vi "Sub_client_v1.vi"() -> ()   [LabVIEW 2019]
uses:
  <vilib>/LabVIEW Open Source Project/MQTT Client/Client class/Client.lvclass/Client.ctl
  <vilib>/LabVIEW Open Source Project/MQTT Connection/MQTT_Base/Base Class/MQTT_Base.lvclass/MQTT_Base.ctl
  <vilib>/LabVIEW Open Source Project/MQTT TCP Connection/MQTT_TCP/Connection/TCPConnection.lvclass
  C:/Program Files (x86)/National Instruments/LabVIEW 2019/vi.lib/LabVIEW Open Source Project/MQTT Connection/MQTT_Connection/Connection/Connection.lvclass
  <vilib>/LabVIEW Open Source Project/MQTT Client/Client class/Client.lvclass
  C:/Program Files (x86)/National Instruments/LabVIEW 2019/vi.lib/LabVIEW Open Source Project/MQTT Connection/MQTT_Base/Base Class/MQTT_Base.lvclass
  <vilib>/LabVIEW Open Source Project/MQTT Control Packets/Control Packets/PUBLISH/PUBLISH.lvclass
  <vilib>/LabVIEW Open Source Project/MQTT Connection/MQTT_Base/Base Class/MQTT_Base.lvclass
panel:
  out "Unsuback":bool
  out "Suback":bool
  in  "Subscribe":bool
  in  "Connection":bool
  in  "Stop Client":bool
  out "Waveform Chart":dbl(graph)
  out "last error":errorcluster
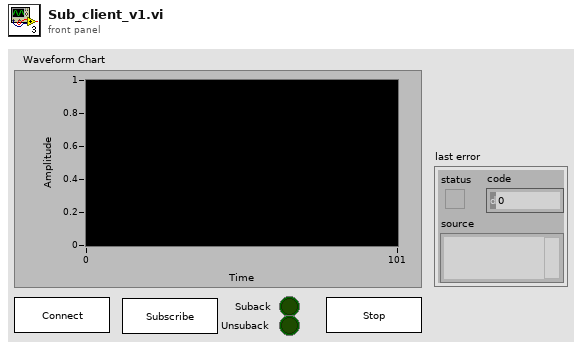
[diagram p1: front panel]
types:
  T1 = typedef "MQTT Client.lvlib/Client.lvclass/Public Events -- cluster.ctl" = cluster{"Connection Status":refnum<user-event>, "Connected":refnum<user-event>, "Application Message":refnum<user-event>}
  T2 = typedef "MQTT Base.lvlib/MQTT_Base.lvclass/Public Events -- cluster.ctl" = cluster{"Stop Event":refnum<user-event>, "Error Event":refnum<user-event>, "Inbound Message":refnum<user-event>}
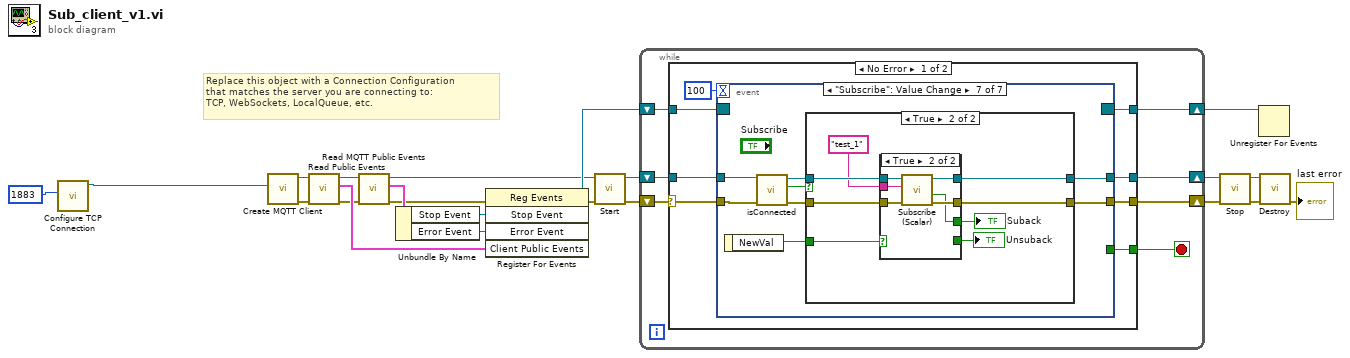
[diagram p0: block diagram]
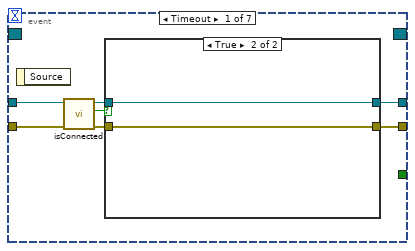
[diagram p2: hidden frame]
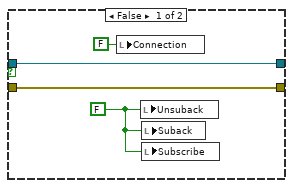
[diagram p3: hidden frame]
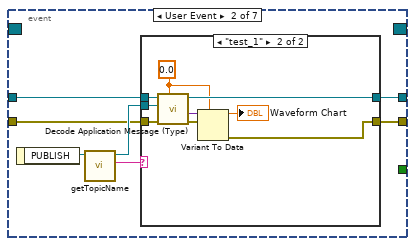
[diagram p4: hidden frame]
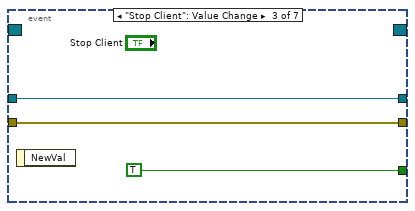
[diagram p6: hidden frame]
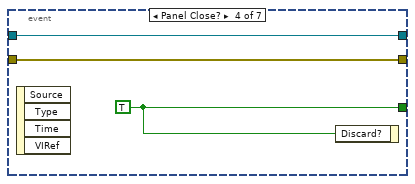
[diagram p7: hidden frame]
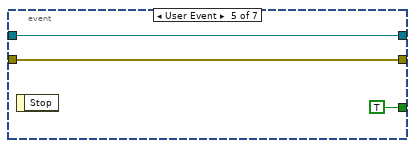
[diagram p8: hidden frame]
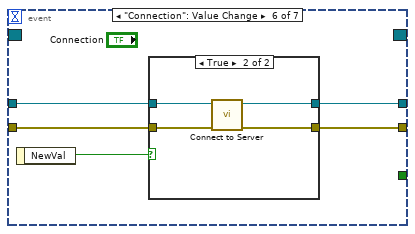
[diagram p9: hidden frame]
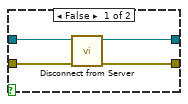
[diagram p10: hidden frame]
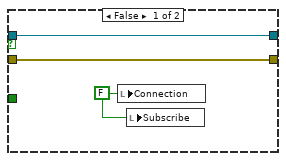
[diagram p11: hidden frame]
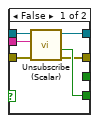
[diagram p12: hidden frame]
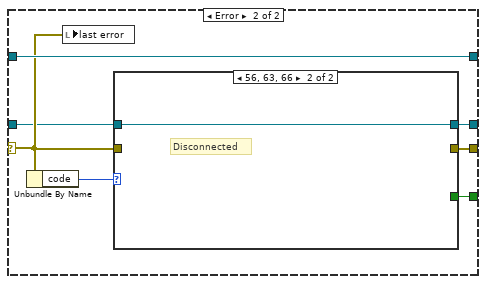
[diagram p13: hidden frame]
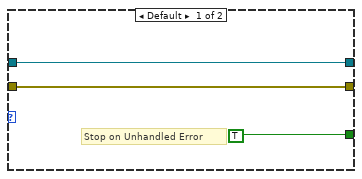
[diagram p14: hidden frame]
diagram:
  # "Replace this object with a Connection Configuration\nthat matches the server you are connecting to:\nTCP, WebSockets, LocalQueue, etc."
  n1 = call <vilib>:"Configure TCP Connection.vi"("remote port (80)"=u16 1883) -> ("TCPConnection"=w1:refnum<class "TCPConnection.lvclass">)  [unwired: 9 in, 1 out]
  n2 = call <vilib>:"Create MQTT Client.vi"("Connection Configuration"=w1) -> ("error out"=w5:errorcluster, "Client out"=w3:refnum<class "Client.lvclass">)  [unwired: 9 in]
  n3 = call <vilib>:"Read Public Events.vi"("error in (no error)"=w5, "Client in"=w3) -> ("error out"=w6:errorcluster, "Client Public Events"=w8:T1, "Client out"=w4:refnum<class "Client.lvclass">)  [unwired: 7 in]
  n4 = call <vilib>:"Read MQTT Public Events.vi"("error in (no error)"=w6, "MQTT_Base in"=w4) -> ("error out"=w7:errorcluster, "MQTT Public Events"=w15:T2, "MQTT_Base out"=w10:refnum<class "Client.lvclass">)  [unwired: 7 in]
  n5 = Unbundle By Name(w15) -> ("Stop Event"=w13:refnum<user-event>, "Error Event"=w14:refnum<user-event>)
  n6 = register-events(error in=w7, w13, w14, w8) -> (reference out=w11:refnum<event-registration>, error out=w9:errorcluster)  [unwired: 1 in]
  n7 = call <vilib>:"Start.vi"("error in (no error)"=w9, "MQTT_Base in"=w10) -> ("error out"=w21:errorcluster, "MQTT_Base out"=w20:refnum<class "Client.lvclass">)  [unwired: 7 in, 1 out]
  n8 = while {
    shift-right: [w28] -> w12
    shift-left: w11 -> [w29]
    shift-right: [w25] -> w17
    shift-left: w20 -> [w26]
    shift-right: [w27] -> w19
    shift-left: w21 -> [w23]
    stop <- w24 stop-if-true
    n9 = case shown="No Error" w23 {
      selector: w23 -> [w30 w125]
      tunnel: w29 -> [w37 w128]
      tunnel: [w36 w128] -> w28
      tunnel: [w35 w123] -> w27
      tunnel: w26 -> [w33 w124]
      tunnel: [w32 w127] -> w25
      tunnel: [w31 w122] -> w24
      frame No Error {
        n10 = event shown="[6] \"Subscribe\": Value Change" {
          selector: w37 -> [_ _ _ _ _ _ _]
          dyn-events: [_ _ _ _ _ _ _] -> w36
          timeout: 100 -> [_ _ _ _ _ _ _]
          tunnel: w30 -> [w40 w54 w70 w72 w77 w78 w96]
          tunnel: [w43 w51 w70 w72 w77 w79 w97] -> w35
          tunnel: [_ _ TRUE w74 TRUE _ _] -> w31
          tunnel: w33 -> [w42 w55 w71 w73 w75 w82 w95]
          tunnel: [w44 w53 w71 w73 w75 w80 w98] -> w32
          event Timeout {
            n11 = event-data() -> ()  [unwired: 1 in, 1 out]
            n12 = call <vilib>:"isConnected.vi"("error in (no error)"=w40, "Client in"=w42) -> ("error out"=w39:errorcluster, "connected"=w38:bool, "Client out"=w41:refnum<class "Client.lvclass">)  [unwired: 7 in]
            n13 = case shown="True" w38 {
              tunnel: [w48 w50] -> w44
              tunnel: [w47 w49] -> w43
              tunnel: w41 -> [w48 w50]
              tunnel: w39 -> [w47 w49]
              frame False {
                w46 = FALSE
                n14 = local write "Connection"(FALSE ("Connection")) -> ()
                n15 = local write "Unsuback"(w46) -> ()
                n16 = local write "Suback"(w46) -> ()
                n17 = local write "Subscribe"(w46) -> ()
              }
              frame True {
              }
            }
          }
          event User Event {
            n18 = event-data() -> ("PUBLISH"=w57:refnum<class "PUBLISH.lvclass">)  [unwired: 1 in]
            n19 = call <vilib>:"getTopicName.vi"("PUBLISH in"=w57) -> ("Topic"=w52:string, "PUBLISH out"=w56:refnum<class "PUBLISH.lvclass">)  [unwired: 8 in, 1 out]
            n20 = case shown="\"test_1\"" w52 {
              tunnel: w56 -> [_ w60]
              tunnel: w55 -> [w59 w66]
              tunnel: w54 -> [w58 w64]
              tunnel: [w59 w65] -> w53
              tunnel: [w58 w68] -> w51
              frame Default {
              }
              frame "test_1" {
                w62 = 0.0
                n21 = call <vilib>:"Decode Application Message (Type).vi"("Type"=w62, "error in (no error)"=w64, "PUBLISH"=w60, "Client in"=w66) -> ("error out"=w63:errorcluster, "Payload"=w61:variant, "Client out"=w65:refnum<class "Client.lvclass">)  [unwired: 4 in, 1 out]
                n22 = Variant To Data(error in=w63, type=w62, Variant=w61) -> (data=→"Waveform Chart":dbl, error out=w68:errorcluster)
              }
            }
          }
          event "Stop Client": Value Change {
            n23 = event-data() -> ()  [unwired: 1 in, 1 out]
          }
          event Panel Close? {
            w74 = TRUE
            n24 = event-data() -> ()  [unwired: 1 in, 4 out]
            n25 = event-data("Discard?"=w74) -> ()  [unwired: 1 in, 1 out]
          }
          event User Event {
            n26 = event-data() -> ()  [unwired: 1 in, 1 out]
          }
          event "Connection": Value Change {
            n27 = event-data() -> ("NewVal"=w81:bool)  [unwired: 1 in]
            n28 = case shown="True" w81 {
              tunnel: w82 -> [w86 w90]
              tunnel: [w85 w87] -> w80
              tunnel: [w84 w88] -> w79
              tunnel: w78 -> [w83 w89]
              frame False {
                n29 = call <vilib>:"Disconnect from Server.vi"("error in (no error)"=w83, "Client in"=w86) -> ("error out"=w84:errorcluster, "Client out"=w85:refnum<class "Client.lvclass">)  [unwired: 7 in, 1 out]
              }
              frame True {
                n30 = call <vilib>:"Connect to Server.vi"("error in (no error)"=w89, "Client in"=w90) -> ("error out"=w88:errorcluster, "Client out"=w87:refnum<class "Client.lvclass">)  [unwired: 6 in, 2 out]
              }
            }
          }
          event "Subscribe": Value Change {
            n31 = event-data() -> ("NewVal"=w91:bool)  [unwired: 1 in]
            n32 = call <vilib>:"isConnected.vi"("error in (no error)"=w96, "Client in"=w95) -> ("error out"=w93:errorcluster, "connected"=w92:bool, "Client out"=w94:refnum<class "Client.lvclass">)  [unwired: 7 in]
            n33 = case shown="True" w92 {
              tunnel: [w101 w109] -> w98
              tunnel: [w100 w108] -> w97
              tunnel: w94 -> [w101 w107]
              tunnel: w93 -> [w100 w106]
              tunnel: w91 -> [_ w104]
              frame False {
                w99 = FALSE ("Connection")
                n34 = local write "Connection"(w99) -> ()
                n35 = local write "Subscribe"(w99) -> ()
              }
              frame True {
                n36 = case shown="True" w104 {
                  tunnel: [w110 w118] -> w109
                  tunnel: [w111 w117] -> w108
                  tunnel: w107 -> [w115 w121]
                  tunnel: w106 -> [w114 w120]
                  tunnel: "test_1" ("Topic Name (empty: Payload name)") -> [w113 w119]
                  tunnel: [_ w116] -> w103
                  tunnel: [w112 _] -> w102
                  frame False {
                    n37 = call <vilib>:"Unsubscribe (Scalar).vi"("error in (no error)"=w114, "Topic Filter"=w113, "Client in"=w115) -> ("error out"=w111:errorcluster, "Ack"=w112:bool, "Client out"=w110:refnum<class "Client.lvclass">)  [unwired: 6 in]
                  }
                  frame True {
                    n38 = call <vilib>:"Subscribe (Scalar).vi"("error in (no error)"=w120, "Topic Filter"=w119, "Client in"=w121) -> ("error out"=w117:errorcluster, "Ack"=w116:bool, "Client out"=w118:refnum<class "Client.lvclass">)  [unwired: 6 in]
                  }
                }
                "Unsuback" <- w102
                "Suback" <- w103
              }
            }
          }
        }
      }
      frame Error {
        n39 = Unbundle By Name(w125) -> ("code"=w126:i32)
        n40 = local write "last error"(w125) -> ()
        n41 = case shown="56, 63, 66" w126 {
          tunnel: w124 -> [w131 w132]
          tunnel: [w131 w132] -> w127
          tunnel: w125 -> [w130 _]
          tunnel: [w130 _] -> w123
          tunnel: [TRUE _] -> w122
          frame Default {
            # "Stop on Unhandled Error"
          }
          frame 56, 63, 66 {
            # "Disconnected"
          }
        }
      }
    }
  }
  n42 = call <vilib>:"Stop.vi"("error in (no error)"=w19, "MQTT_Base in"=w17) -> ("error out"=w18:errorcluster, "MQTT_Base out"=w16:refnum<class "Client.lvclass">)  [unwired: 7 in, 1 out]
  n43 = Unregister For Events(event registration refnum=w12) -> ()  [unwired: 1 in, 1 out]
  n44 = call <vilib>:"Destroy.vi"("error in (no error)"=w18, "MQTT_Base in"=w16) -> ("error out"=→"last error":errorcluster)  [unwired: 8 in, 1 out]
